vi "UPS配置同步 (子VI).vi"(11 "Boolean输入":refnum<vi>) -> ()   [LabVIEW 2016, in "环境动力监测库.lvlib" / "UPS库.lvlib"]
uses:
  <vilib>/Utility/config.llb/NI_LVConfig.lvlib
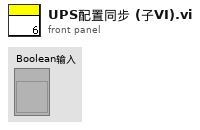
[diagram p1: front panel]
types:
  T1 = cluster{"枚举":enum16{"open", "read", "write", "close"}, "写入缓冲区":string}
  T2 = enum16{"山特UPSC1~3", "山特UPSC6~20", "华为UPS2000-G-(1-3KVA)"}
  T3 = cluster{"监测项描述:输出":string, "连接方式":enum16{"串口", "TCP"}, "端口":string, "IP address:":string, "Port:":string, "站号":u64, "传感器型号":string, "波特率":u64, "data bits":u64, "停止位":u16, "奇偶校验":u16}
  T4 = typedef "NI_LVConfig.lvlib/Config Data RefNum.ctl" = refnum<k1>
  T5 = cluster{"VISA resource name":refnum<visa-resource-name>, "Serial Config":cluster{"baud rate (9600)":u32, "stop bits (10: 1 bit)":u16, "parity (0:none)":enum16{"None", "Odd", "Even", "Mark", "Space"}, "data bits (8)":u16, "timeout (10sec)":u32}, "型号选择":enum16{"山特UPSC1~3", "山特UPSC6~20", "华为UPS2000-G-(1-3KVA)"}, "HW-UPS-2000 MB session":refnum<class "MB_Master.lvclass">, "连接方式":enum16{"串口", "TCP"}, "IP":string, "Port":string}
  T6 = cluster{"baud rate (9600)":u32, "stop bits (10: 1 bit)":u16, "parity (0:none)":enum16{"None", "Odd", "Even", "Mark", "Space"}, "data bits (8)":u16, "timeout (10sec)":u32}
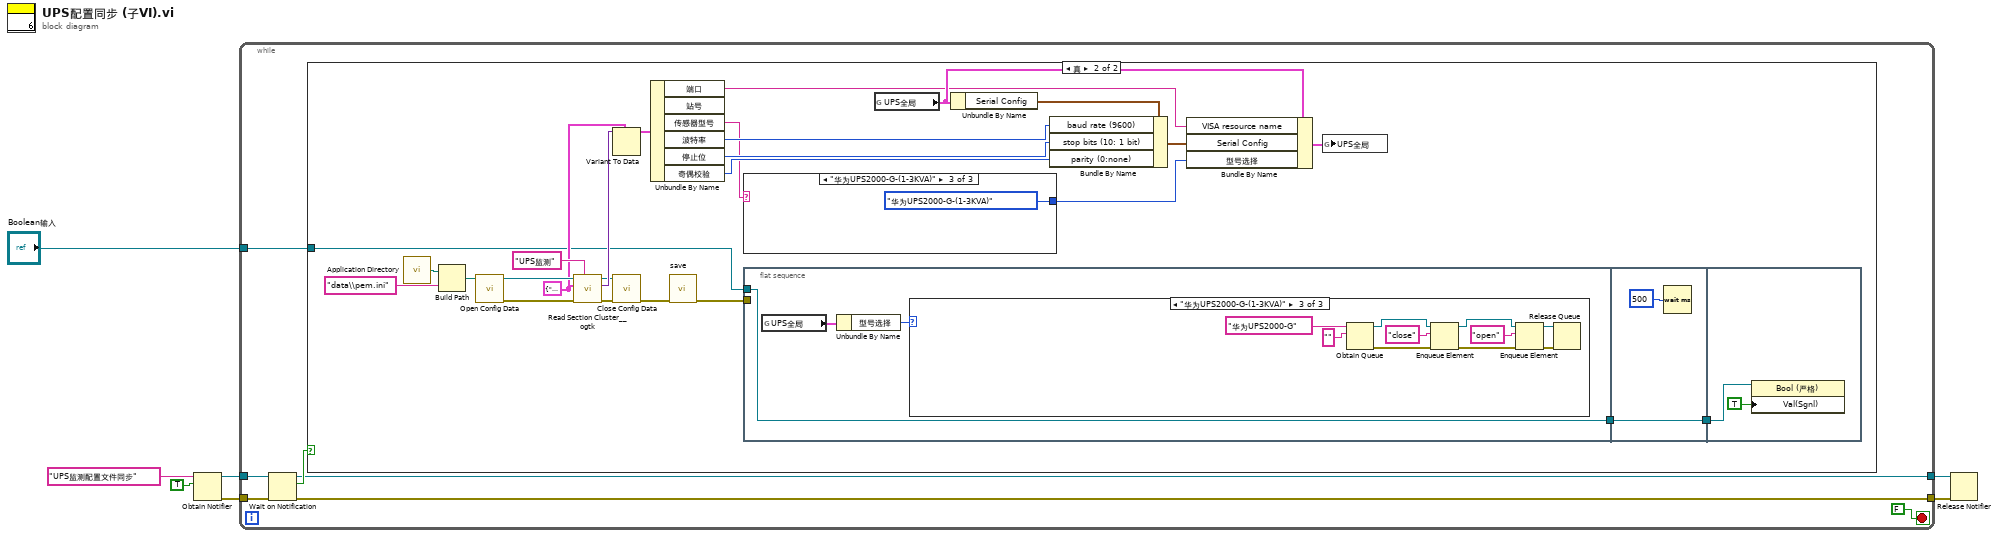
[diagram p0: block diagram]
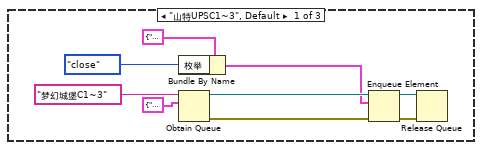
[diagram p3: hidden frame]
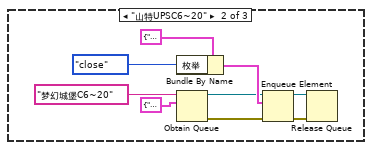
[diagram p4: hidden frame]
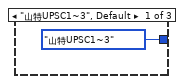
[diagram p5: hidden frame]
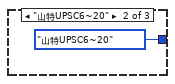
[diagram p6: hidden frame]
diagram:
  n1 = Obtain Notifier(name (unnamed)="UPS监测配置文件同步" ("名称（未命名）"), notification data type=TRUE) -> (notifier out=w4:refnum<notifier>, error out=w5:errorcluster)  [unwired: 2 in, 1 out]
  n2 = while {
    tunnel: w4 -> [w14]
    tunnel: w5 -> [w13]
    tunnel: [w10] -> w6
    tunnel: [w9] -> w7
    tunnel: "Boolean输入" -> [w8]
    stop <- FALSE stop-if-true
    n3 = Wait on Notification(notifier=w14, error in (no error)=w13) -> (notifier out=w10:refnum<notifier>, notification=w12:bool, error out=w9:errorcluster)  [unwired: 2 in, 1 out]
    n4 = case shown="真" w12 {
      tunnel: w8 -> [_ w25]
      frame False {
      }
      frame True {
        w26 = T3 {"监测项描述:输出"="", "连接方式"=enum."串口", "端口"="", "IP address:"="", "Port:"="", "站号"=19200, "传感器型号"="", "波特率"=19200, "data bits"=8, "停止位"=10, "奇偶校验"=0} ("输入簇")
        n5 = call <vilib>:"Application Directory.vi"() -> ("Application Directory"=w30:path)
        n6 = Build Path(base path=w30, name or relative path="data\\pem.ini" ("名称或相对路径")) -> (appended path=w29:path)
        n7 = call <vilib>:"Open Config Data.vi"("configuration file path"=w29) -> ("error out"=w28:errorcluster, "refnum"=w27:T4)  [unwired: 8 in, 1 out]
        n8 = call <userlib>:"Read Section Cluster__ogtk.vi"("section (optional)"="UPS监测", "error in (no error)"=w28, "Section Formatted Cluster Type"=w26, "refnum"=w27) -> ("error out"=w34:errorcluster, "Section Formatted Cluster"=w35:variant, "dup refnum"=w33:T4)  [unwired: 3 in, 2 out]
        n9 = Variant To Data(type=w26, Variant=w35) -> (data=w36:T3)  [unwired: 1 in, 1 out]
        n10 = call <vilib>:"Close Config Data.vi"("error in (no error)"=w34, "refnum"=w33) -> ("error out"=w22:errorcluster)  [unwired: 8 in, 1 out]
        n11 = Unbundle By Name(w36) -> ("端口"=w19:string, "传感器型号"=w37:string, "波特率"=w38:u64, "停止位"=w39:u16, "奇偶校验"=w40:u16)  [unwired: 1 out]
        n12 = call "save.vi"("error in (no error)"=w22) -> ("error out"=w21:errorcluster)  [unwired: 10 in]
        n13 = case shown="\"华为UPS2000-G-(1-3KVA)\"" w37 {
          tunnel: [T2."山特UPSC1~3" ("型号选择") T2."山特UPSC6~20" ("型号选择") T2."华为UPS2000-G-(1-3KVA)" ("型号选择")] -> w16
          frame "山特UPSC1~3", Default {
          }
          frame "山特UPSC6~20" {
          }
          frame "华为UPS2000-G-(1-3KVA)" {
          }
        }
        n14 = flat-sequence {
          tunnel: w25 -> [w43]
          tunnel: [w43] -> w23
          tunnel: w21 -> [_]
          tunnel: [w72] -> w24
          tunnel: w23 -> [w72]
          tunnel: w24 -> [w74]
          frame #0 {
            n15 = global read "断电保存全局变量.vi" "UPS全局"() -> (w42:T5)
            n16 = Unbundle By Name(w42) -> ("型号选择"=w41:T2)
            n17 = case shown="\"华为UPS2000-G-(1-3KVA)\"" w41 {
              frame "山特UPSC1~3", Default {
                n18 = Bundle By Name(cluster=T1 {"枚举"=enum."open", "写入缓冲区"=""}, "枚举"=enum16{"open", "read", "write", "close"}."close") -> (w46:T1)
                n19 = Obtain Queue(name (unnamed)="梦幻城堡C1~3" ("名称（未命名）"), element data type=T1 {"枚举"=enum."open", "写入缓冲区"=""}) -> (queue out=w49:refnum<queue>, error out=w50:errorcluster)  [unwired: 3 in, 1 out]
                n20 = Enqueue Element(queue=w49, element=w46, error in (no error)=w50) -> (queue out=w51:refnum<queue>, error out=w52:errorcluster)  [unwired: 1 in, 1 out]
                n21 = Release Queue(queue=w51, error in (no error)=w52) -> ()  [unwired: 1 in, 3 out]
              }
              frame "山特UPSC6~20" {
                n22 = Bundle By Name(cluster=T1 {"枚举"=enum."open", "写入缓冲区"=""}, "枚举"=enum16{"open", "read", "write", "close"}."close" ("元素")) -> (w57:T1)
                n23 = Obtain Queue(name (unnamed)="梦幻城堡C6~20" ("名称（未命名）"), element data type=T1 {"枚举"=enum."open", "写入缓冲区"=""}) -> (queue out=w56:refnum<queue>, error out=w55:errorcluster)  [unwired: 3 in, 1 out]
                n24 = Enqueue Element(queue=w56, element=w57, error in (no error)=w55) -> (queue out=w54:refnum<queue>, error out=w53:errorcluster)  [unwired: 1 in, 1 out]
                n25 = Release Queue(queue=w54, error in (no error)=w53) -> ()  [unwired: 1 in, 3 out]
              }
              frame "华为UPS2000-G-(1-3KVA)" {
                n26 = Obtain Queue(name (unnamed)="华为UPS2000-G" ("名称（未命名）"), element data type="") -> (queue out=w66:refnum<queue>, error out=w65:errorcluster)  [unwired: 3 in, 1 out]
                n27 = Enqueue Element(queue=w66, element="close" ("元素"), error in (no error)=w65) -> (queue out=w63:refnum<queue>, error out=w62:errorcluster)  [unwired: 1 in, 1 out]
                n28 = Enqueue Element(queue=w63, element="open" ("元素"), error in (no error)=w62) -> (queue out=w70:refnum<queue>, error out=w71:errorcluster)  [unwired: 1 in, 1 out]
                n29 = Release Queue(queue=w70, error in (no error)=w71) -> ()  [unwired: 1 in, 3 out]
              }
            }
          }
          frame #1 {
            n30 = Wait (ms)(milliseconds to wait=u32 500 ("等待时间（毫秒）")) -> ()  [unwired: 1 out]
          }
          frame #2 {
            n31 = property on="属性节点" class="Bool (严格)"(reference=w74, "Val(Sgnl)"=TRUE) -> ()  [unwired: 1 in, 2 out]
          }
        }
        n32 = global read "断电保存全局变量.vi" "UPS全局"() -> (w20:T5)
        n33 = Unbundle By Name(w20) -> ("Serial Config"=w18:T6)
        n34 = Bundle By Name(cluster=w18, "baud rate (9600)"=w38, "stop bits (10: 1 bit)"=w39, "parity (0:none)"=w40) -> (w17:T6)
        n35 = Bundle By Name(cluster=w20, "VISA resource name"=w19, "Serial Config"=w17, "型号选择"=w16) -> (w15:T5)
        n36 = global write "断电保存全局变量.vi" "UPS全局"(w15) -> ()
      }
    }
  }
  n37 = Release Notifier(notifier=w6, error in (no error)=w7) -> ()  [unwired: 1 in, 3 out]
